vi "CheckMaxNumFiles.vi"(6 "Qbus":refnum<class "Qbus.lvclass">, 8 "error in (no error)":errorcluster, 9 "data":T1, 10 "data event config":T6, 11 "config":T5) -> (0 "error out":errorcluster, 3 "ok to open new file":bool)   [LabVIEW 2017, in "CmsDataEventCreator.lvlib"]
uses:
  <vilib>/addons/InsightCM/Devices/Shared/Cms/CmsDataEventCreator/CmsDataEventCreator.lvlib
  <vilib>/addons/InsightCM/Devices/Shared/Cms/CmsDataEventCreator/controls/DataEventConfig.ctl
  <vilib>/addons/InsightCM/Devices/Shared/Cms/CmsDataEventCreator/controls/AcqParams.ctl
  <vilib>/addons/InsightCM/Devices/Shared/Common/DataAccumulator/controls/AccumulationSettings.ctl
  <vilib>/addons/InsightCM/Devices/Shared/Common/DataAccumulator/controls/accumulationType.ctl
  <vilib>/addons/InsightCM/Devices/Shared/Common/DVRBuffer/controls/BufferLocation.ctl
  <vilib>/addons/PointValueMap/controls/PointMap.ctl
  <vilib>/addons/InsightCM/Devices/Shared/Cms/CmsDataEventCreator/controls/config.ctl
  <vilib>/addons/InsightCM/Devices/Shared/Common/DataFlow/controls/Data.ctl
  <vilib>/addons/InsightCM/Utilities/DataAccessors/controls/wfmSGL_DVR.ctl
  <vilib>/addons/InsightCM/Devices/Shared/Common/DataFlow/controls/Type.ctl
  <vilib>/addons/Qbus/Qbus.lvclass
  <vilib>/addons/PointValueMap/PointValueMap.lvlib
  <vilib>/addons/InsightCM/Devices/Shared/Common/DVRBuffer/DVRBuffer.lvlib
  <vilib>/addons/InsightCM/Devices/Shared/Common/DataAccumulator/DataAccumulator.lvlib
  <vilib>/addons/InsightCM/Devices/Shared/Common/DataFlow/DataFlow.lvlib
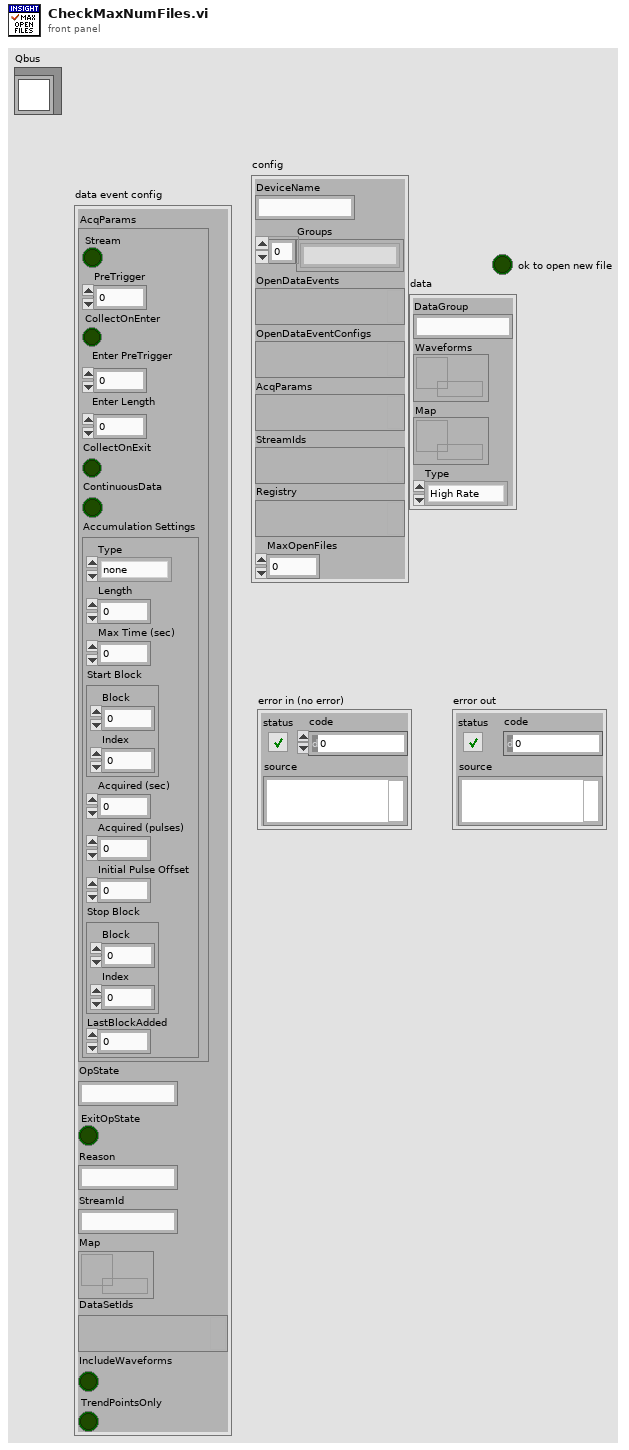
[diagram p1: front panel]
types:
  T1 = typedef "DataFlow.lvlib/Data.ctl" = cluster{"DataGroup":string, "Waveforms":T2, "Map":T3, "Type":T4}
  T2 = typedef "wfmSGL_DVR.ctl" = refnum<data-value>
  T3 = typedef "PointValueMap.lvlib/PointMap.ctl" = refnum<data-value>
  T4 = typedef "DataFlow.lvlib/Type.ctl" = enum16{"High Rate", "Low Rate", "Burst Mode"}
  T5 = typedef "CmsDataEventCreator.lvlib/config.ctl" = cluster{"DeviceName":string, "Groups":string[], "OpenDataEvents":variant, "OpenDataEventConfigs":variant, "AcqParams":variant, "StreamIds":variant, "Registry":variant, "MaxOpenFiles":i32}
  T6 = typedef "CmsDataEventCreator.lvlib/DataEventConfig.ctl" = cluster{"AcqParams":T7, "OpState":string, "ExitOpState":bool, "Reason":string, "StreamId":string, "Map":T3, "DataSetIds":variant, "IncludeWaveforms":bool, "TrendPointsOnly":bool}
  T7 = typedef "CmsDataEventCreator.lvlib/AcqParams.ctl" = cluster{"Stream":bool, "PreTrigger":i32, "CollectOnEnter":bool, "Enter PreTrigger":i32, "Enter Length":dbl, "CollectOnExit":bool, "ContinuousData":bool, "Accumulation Settings":T8}
  T8 = typedef "DataAccumulator.lvlib/AccumulationSettings.ctl" = cluster{"Type":T9, "Length":dbl, "Max Time (sec)":dbl, "Start Block":T10, "Acquired (sec)":dbl, "Acquired (pulses)":i32, "Initial Pulse Offset":dbl, "Stop Block":T10, "LastBlockAdded":u32}
  T9 = typedef "DataAccumulator.lvlib/accumulationType.ctl" = enum16{"none", "seconds", "revolutions"}
  T10 = typedef "DVRBuffer.lvlib/BufferLocation.ctl" = cluster{"Block":u32, "Index":i32}
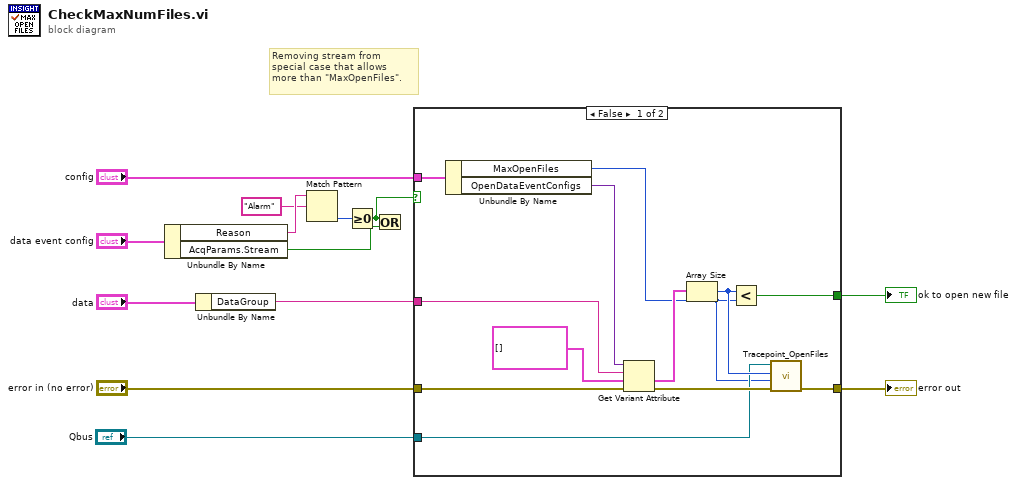
[diagram p0: block diagram]
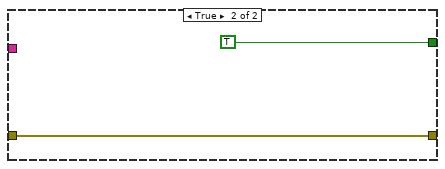
[diagram p2: hidden frame]
diagram:
  # "Removing stream from\nspecial case that allows\nmore than \"MaxOpenFiles\"."
  n1 = Unbundle By Name("data event config") -> ("Reason"=w7:string, "AcqParams.Stream"=w8:bool)
  n2 = Unbundle By Name("data") -> ("DataGroup"=w3:string)
  n3 = Match Pattern(string=w7, regular expression="Alarm" ("x")) -> (offset past match=w5:i32)  [unwired: 1 in, 3 out]
  n4 = Greater Or Equal To 0?(x=w5) -> (x >= 0?=w2:bool)
  n5 = Or(x=w2, y=w8) -> ()  [unwired: 1 out]
  n6 = case shown="False" w2 {
    tunnel: [w16 w27] -> w12
    tunnel: "error in (no error)" -> [w24 w27]
    tunnel: [w20 TRUE ("ok to open new file")] -> w10
    tunnel: "config" -> [w23 _]
    tunnel: w3 -> [w19 _]
    tunnel: "Qbus" -> [w15 _]
    frame False {
      n7 = Unbundle By Name(w23) -> ("MaxOpenFiles"=w14:i32, "OpenDataEventConfigs"=w22:variant)
      n8 = Get Variant Attribute(Variant=w22, name=w19, default value (empty Variant)=T6[] [], error in=w24) -> (value=w21:T6[], error out=w17:errorcluster)  [unwired: 2 out]
      n9 = Array Size(array=w21) -> (size(s)=w18:i32)
      n10 = Less?(x=w18, y=w14) -> (x < y?=w20:bool)
      n11 = call <vilib>:"Tracepoint_OpenFiles.vi"("error in (no error)"=w17, "max open files"=w14, "open files"=w18, "Qbus"=w15) -> ("error out"=w16:errorcluster)  [unwired: 7 in]
    }
    frame True {
    }
  }
  "ok to open new file" <- w10
  "error out" <- w12
